vi "ConvertFromConfigurationFile.vi"() -> ()   [LabVIEW 2017]
panel:
  out "values":string[](array[string])
  out "keys":string[](array[string])
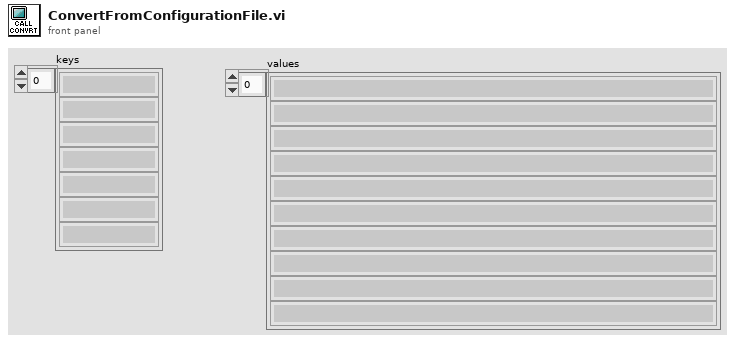
[diagram p1: front panel]
types:
  T1 = enum16{"open", "replace", "create", "open or create", "replace or create", "replace or create with confirmation"}
  T2 = cluster{"Files to Preload":path[], "File(s)/Folder to convert":path, "Destination Folder (relative to output path)":path}
  T3 = cluster{"Files to Preload":path[], "File(s)/Folder to convert":path, "Destination Folder (relative to output path)":path}[]
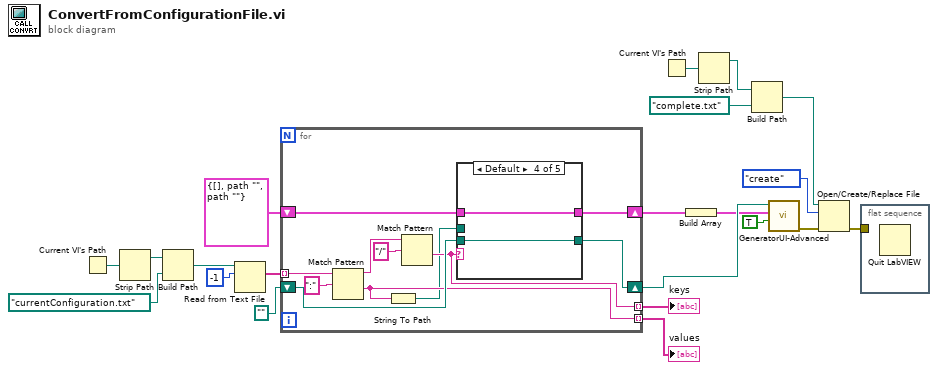
[diagram p0: block diagram]
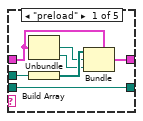
[diagram p2: hidden frame]
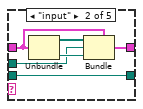
[diagram p3: hidden frame]
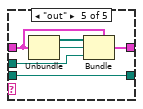
[diagram p5: hidden frame]
diagram:
  n1 = Current VI's Path() -> (path=w8:path)
  n2 = Strip Path(path=w8) -> (stripped path=w7:path)  [unwired: 1 out]
  n3 = Build Path(base path=w7, name or relative path=path "currentConfiguration.txt" ("file (use dialog)")) -> (appended path=w5:path)
  n4 = Read from Text File(file (use dialog)=w5, count=-1) -> (text=w13:string[])  [unwired: 2 in, 3 out]
  n5 = for {
    tunnel: w13 -> [w31] mode=indexing
    shift-right: [w28] -> w21
    shift-left: path "" -> [w27]
    shift-right: [w26] -> w18
    shift-left: T2 {"Files to Preload"=[], "File(s)/Folder to convert"=path "", "Destination Folder (relative to output path)"=path ""} ("ConversionFiles") -> [w25]
    tunnel: [w24] -> w15 mode=indexing
    tunnel: [w23] -> w14 mode=indexing
    n6 = Match Pattern(string=w31, regular expression=":") -> (before substring=w30:string, after substring=w23:string)  [unwired: 1 in, 2 out]
    n7 = String To Path(string=w23) -> (path=w22:path)
    n8 = Match Pattern(string=w30, regular expression="/") -> (after substring=w24:string)  [unwired: 1 in, 3 out]
    n9 = case shown="Default" w24 {
      tunnel: [w39 w43 w46 w49 w52] -> w28
      tunnel: w27 -> [w39 w43 _ w49 w52]
      tunnel: [w38 w42 w47 w48 w54] -> w26
      tunnel: w25 -> [w34 w41 w47 w48 w51]
      tunnel: w22 -> [w33 w40 w46 _ w50]
      frame "preload" {
        n10 = Unbundle(w34) -> ("File(s)/Folder to convert"=w36:path, "Destination Folder (relative to output path)"=w35:path)  [unwired: 1 out]
        n11 = Build Array(w33) -> (w37:path[])
        n12 = Bundle(cluster=w34, "Files to Preload"=w37, "File(s)/Folder to convert"=w36, "Destination Folder (relative to output path)"=w35) -> (w38:T2)
      }
      frame "input" {
        n13 = Unbundle(w41) -> ("Files to Preload"=w45:path[], "Destination Folder (relative to output path)"=w44:path)  [unwired: 1 out]
        n14 = Bundle(cluster=w41, "Files to Preload"=w45, "File(s)/Folder to convert"=w40, "Destination Folder (relative to output path)"=w44) -> (w42:T2)
      }
      frame "top" {
      }
      frame Default {
      }
      frame "out" {
        n15 = Unbundle(w51) -> ("Files to Preload"=w53:path[], "File(s)/Folder to convert"=w55:path)  [unwired: 1 out]
        n16 = Bundle(cluster=w51, "Files to Preload"=w53, "File(s)/Folder to convert"=w55, "Destination Folder (relative to output path)"=w50) -> (w54:T2)
      }
    }
  }
  "keys" <- w15
  "values" <- w14
  n17 = Current VI's Path() -> (path=w4:path)
  n18 = Build Array(w18) -> (w20:T3)
  n19 = Strip Path(path=w4) -> (stripped path=w3:path)  [unwired: 1 out]
  n20 = Build Path(base path=w3, name or relative path=path "complete.txt" ("file (use dialog)")) -> (appended path=w1:path)
  n21 = call "GeneratorUI-Advanced.vi"("Unattended Mode"=TRUE, "File configurations"=w20, "Top level output path"=w21) -> ("error out"=w10:errorcluster)  [unwired: 8 in]
  n22 = Open/Create/Replace File(file path (use dialog)=w1, error in=w10, operation (0:open)=T1."create") -> (error out=w9:errorcluster)  [unwired: 3 in, 2 out]
  n23 = flat-sequence {
    tunnel: w9 -> [_]
    frame #0 {
      n24 = Quit LabVIEW() -> ()  [unwired: 1 in]
    }
  }
